vi "setUp.vi"(8 "error in":errorcluster, 11 "reference in":refnum<class "Logging Loopback.lvclass">) -> (0 "error out":errorcluster, 3 "reference out":refnum<class "Logging Loopback.lvclass">)   [LabVIEW 2020, in "Logging Loopback.lvclass"]
doc: "setUp runs prior to the test method during test execution. Use this method to initialize any object data required by your tests."
uses:
  Logging Loopback.lvclass
  C:/Program Files (x86)/National Instruments/LabVIEW 2020/vi.lib/addons/_JKI Toolkits/VI Tester/TestCase.llb/TestCase.lvclass
  Logging Loopback.lvclass/Logging Loopback.ctl
  <vilib>/addons/_JKI Toolkits/VI Tester/TestCase.llb/TestCase.lvclass
  niveristand-custom-device-testing-tools/VeriStandTestUtilities/VeriStandTestUtilities.lvlib
  <vilib>/WebDAVClient/NI_WebDAV.lvlib
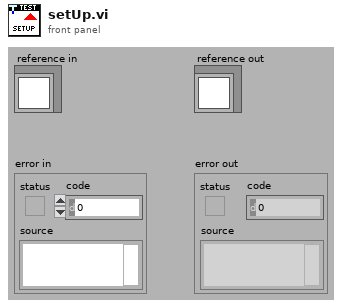
[diagram p1: front panel]
types:
  T1 = typedef "Custom Device API.lvlib/Custom Device Item Ref.ctl" = u64
  T2 = typedef "NI_WebDAV.lvlib/SessionHandle.ctl" = refnum<k1>
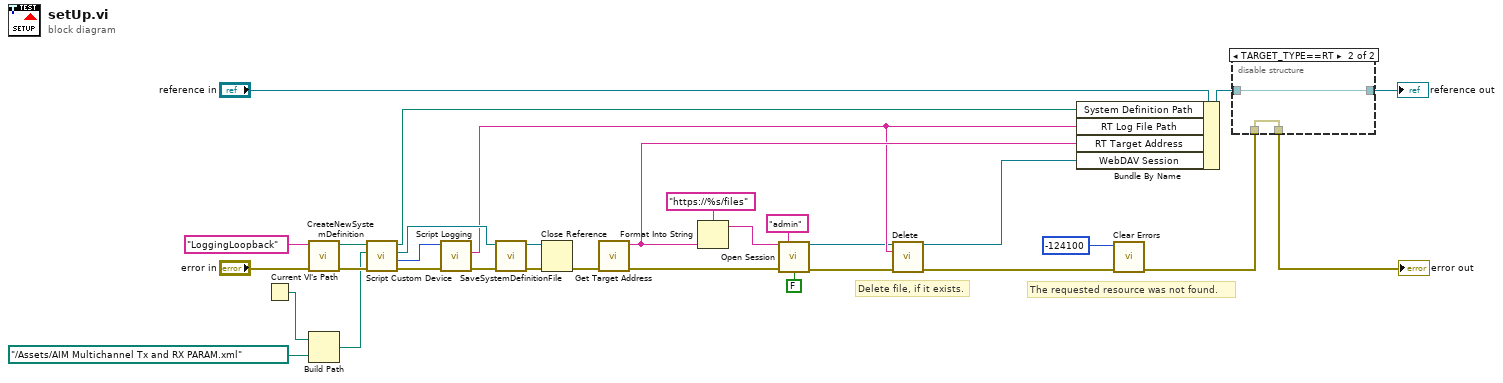
[diagram p0: block diagram]
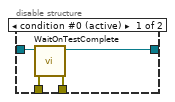
[diagram p2: hidden frame]
diagram:
  # "Delete file, if it exists."
  # "The requested resource was not found."
  n1 = Current VI's Path() -> (path=w16:path)
  n2 = call "CreateNewSystemDefinition.vi"("error in"="error in", "System Definition Name"="LoggingLoopback" ("Channel")) -> ("error out"=w27:errorcluster, "System Definition Path"=w26:path)  [unwired: 8 in]
  n3 = Build Path(base path=w16, name or relative path=path "../Assets/AIM Multichannel Tx and RX PARAM.xml" ("Hardware File Path")) -> (appended path=w7:path)
  n4 = call "Script Custom Device.vi"("error in"=w27, "Parameter File Path"=w7, "System Definition File Path In"=w26) -> ("error out"=w23:errorcluster, "AIM ARINC 429 custom device out"=w22:T1, "System Definition Reference"=w25:refnum<k24>, "System Definition File Path Out"=w10:path)  [unwired: 5 in]
  n5 = call "Script Logging.vi"("error in (no error)"=w23, "Ballard ARINC 429 custom device in"=w22) -> ("error out"=w21:errorcluster, "RT log file path"=w13:string)  [unwired: 7 in, 1 out]
  n6 = call "SaveSystemDefinitionFile.vi"("error in (no error)"=w21, "System Definition Reference in"=w25) -> ("error out"=w20:errorcluster, "System Definition Reference out"=w19:refnum<k24>)  [unwired: 8 in]
  n7 = Close Reference(reference=w19, error in (no error)=w20) -> (error out=w17:errorcluster)
  n8 = call "Get Target Address.vi"("error in (no error)"=w17) -> ("error out"=w15:errorcluster, "target address"=w14:string)  [unwired: 9 in]
  n9 = Format Into String(format string="https://%s/files" ("host uri prefix"), w14) -> (resulting string=w2:string)  [unwired: 2 in, 1 out]
  n10 = call <vilib>:"Open Session.vi"("host uri prefix"=w2, "username"="admin", "error in (no error)"=w15, "verify server?"=FALSE) -> ("session handle out"=w6:T2, "error out"=w5:errorcluster)  [unwired: 10 in]
  n11 = call <vilib>:"Delete.vi"("session handle"=w6, "relative uri"=w13, "error in (no error)"=w5) -> ("session handle out"=w8:T2, "error out"=w12:errorcluster)  [unwired: 11 in]
  n12 = Bundle By Name(cluster="reference in", "System Definition Path"=w10, "RT Log File Path"=w13, "RT Target Address"=w14, "WebDAV Session"=w8) -> (w18:refnum<class "Logging Loopback.lvclass">)
  n13 = call <vilib>:"Clear Errors.vi"("error in (no error)"=w12, "specific error code to clear (0: all)"=-124100) -> ("error out"=w9:errorcluster)  [unwired: 4 in, 1 out]
  n14 = disable-structure shown="TARGET_TYPE==RT" {
    disable-tunnel: w9 -> [w36 w37]
    disable-tunnel: [w35 w37] -> w32
    disable-tunnel: [w34 w38] -> w30
    disable-tunnel: w18 -> [w33 w38]
    frame condition #0 (active) {
      n15 = call <vilib>:"WaitOnTestComplete.vi"("error in (no error)"=w36, "TestCase in"=w33) -> ("error out"=w35:errorcluster, "TestCase out"=w34:refnum<class "Logging Loopback.lvclass">)  [unwired: 8 in]
    }
    frame condition #1 {
    }
  }
  "error out" <- w32
  "reference out" <- w30
